vi "Echo QDFunctions.vi"(0 "QDFunction in":refnum<class "QDList.lvclass">, 1 "Shift Pressed?":bool, 5 "QD Launch VI Ref":refnum<vi>, 7 "QD Combo Box Ref":refnum<vi>, 9 "QDFunction":string, 11 "error in (no error)":errorcluster, 12 "Variant in":variant) -> (4 "QDFunction out":refnum<class "QDList.lvclass">, 15 "error out":errorcluster)   [LabVIEW 2015, in "QDList.lvclass"]
uses:
  QDList.lvclass
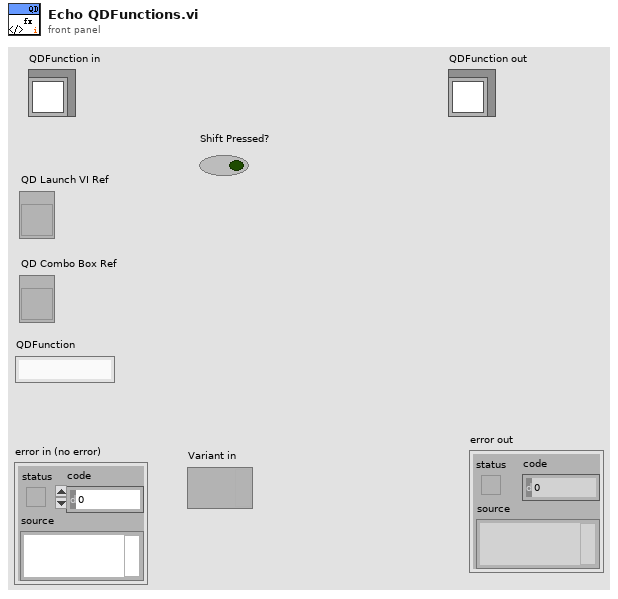
[diagram p1: front panel]
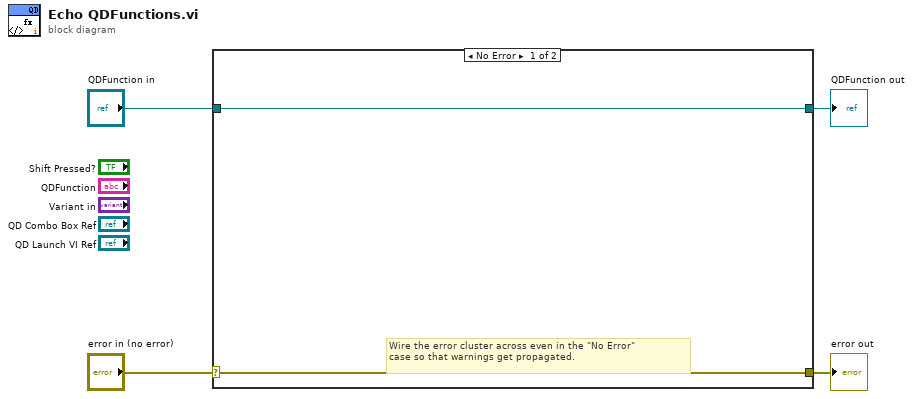
[diagram p0: block diagram]
diagram:
  n1 = case shown="No Error" "error in (no error)" {
    selector: "error in (no error)" -> [w5 w8]
    tunnel: [w5 w8] -> w3
    tunnel: [w6 w7] -> w1
    tunnel: "QDFunction in" -> [w6 w7]
    frame No Error {
      # "Wire the error cluster across even in the \"No Error\"\ncase so that warnings get propagated."
    }
    frame Error {
    }
  }
  "error out" <- w3
  "QDFunction out" <- w1
